vi "Machine - Config File.vi"(5 "Setting":bool, 6 "Action":enum16{"Write", "Read", "Read All", "Remove"}(ring), 7 "V1":bool, 8 "error in (no error)":errorcluster, 9 "Value":string[](array[string]), 10 "Key Name":string[](array[string]), 11 "IP/SN":string) -> (0 "error out":errorcluster, 3 "Value Out":cluster{"IP/SN":string, "Key Value":string[]}[](array[cluster]))   [LabVIEW 2019]
uses:
  <vilib>/Utility/config.llb/Write Key (String).vi
  <vilib>/Utility/config.llb/Read Key (String).vi
  <vilib>/httpClient/POSTBuffer.vi
  <vilib>/Utility/config.llb/NI_LVConfig.lvlib
  <vilib>/httpClient/LabVIEWHTTPClient.lvlib
panel:
  out "?":cluster{"IP/SN":string, "Key Value":string[]}={"IP/SN"="TP2-240203", "Key Value"=["COM6", "TEST2", "0", "N/A"]}
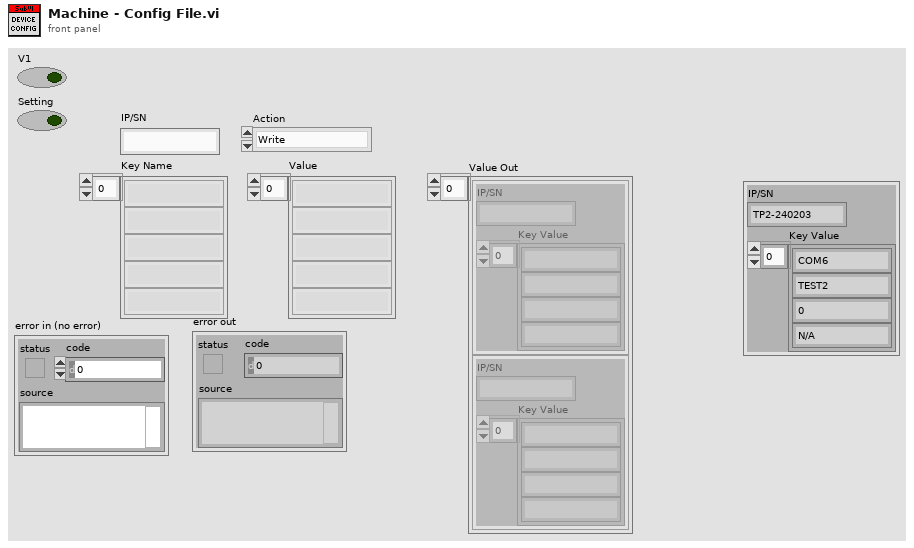
[diagram p1: front panel]
types:
  T1 = cluster{"action":string, "SNIP":string, "port":string, "devicename":string, "status":string, "type":string, "id":string}
  T2 = cluster{"IP Address":string, "Key Value":string[]}
  T3 = cluster{"status":string, "data":cluster{"SNIP":string, "port":string, "devicename":string, "status":string, "type":string, "delete":string, "id":string}[]}
  T4 = cluster{"action":string, "SNIP":string, "port":string, "devicename":string, "status":string, "type":string}
  T5 = typedef "NI_LVConfig.lvlib/Config Data RefNum.ctl" = refnum<k1>
  T6 = typedef "LabVIEWHTTPClient.lvlib/ClientHandle.ctl" = refnum<k1>
  T7 = cluster{"SNIP":string, "port":string, "devicename":string, "status":string, "type":string, "delete":string, "id":string}[]
  T8 = cluster{"SNIP":string, "port":string, "devicename":string, "status":string, "type":string, "delete":string, "id":string}
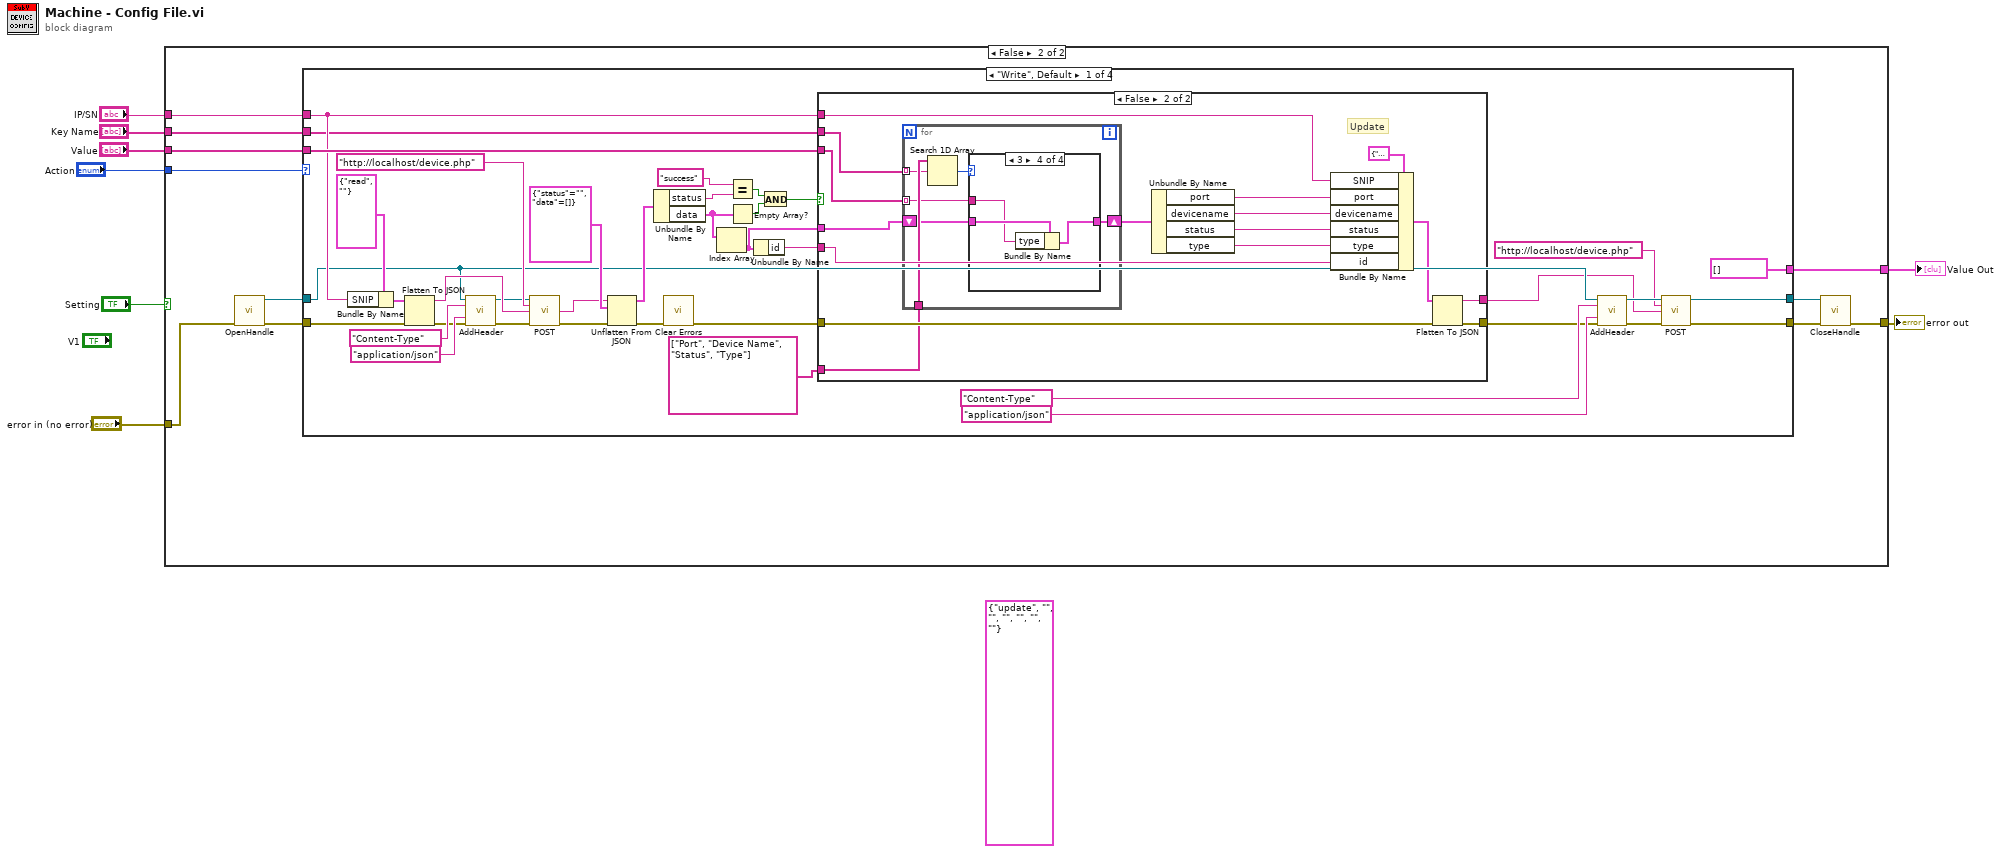
[diagram p0: block diagram]
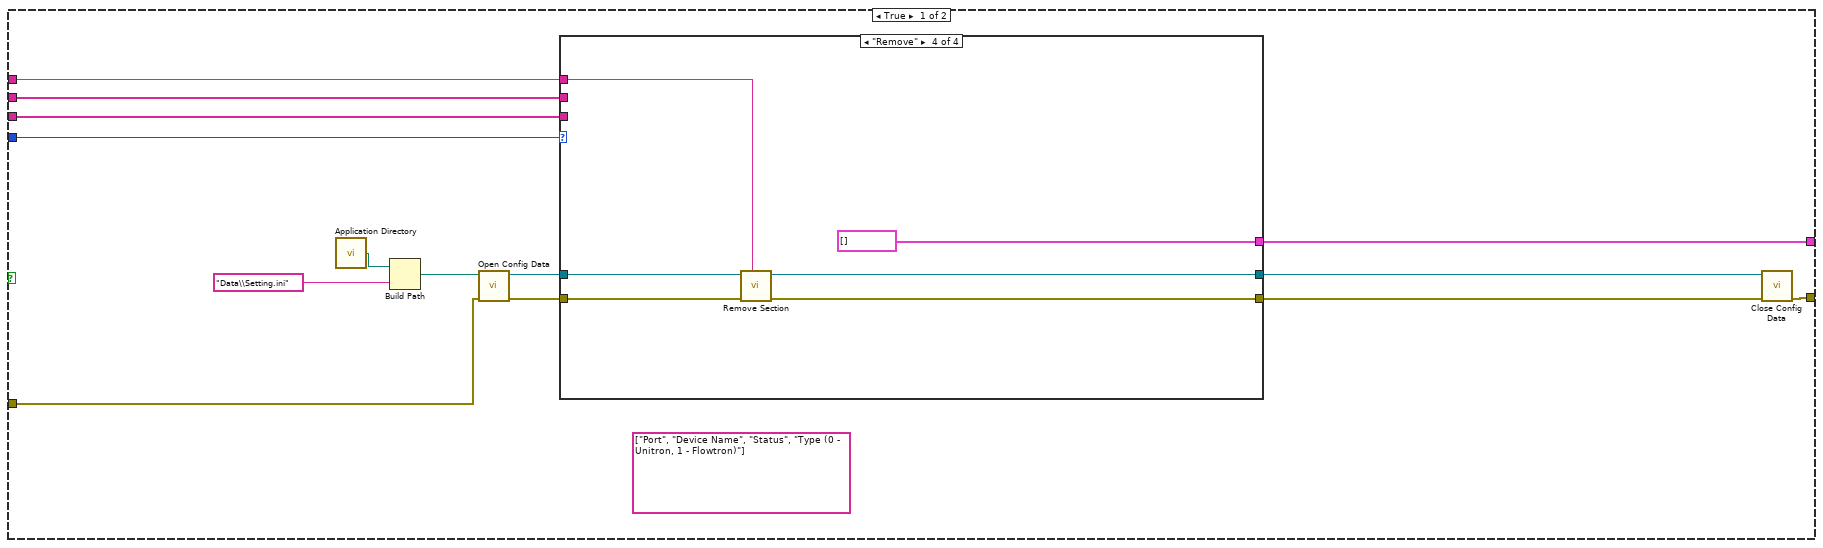
[diagram p2: hidden frame]
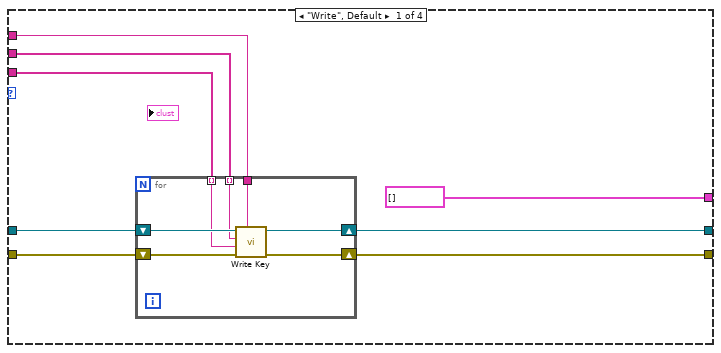
[diagram p3: hidden frame]
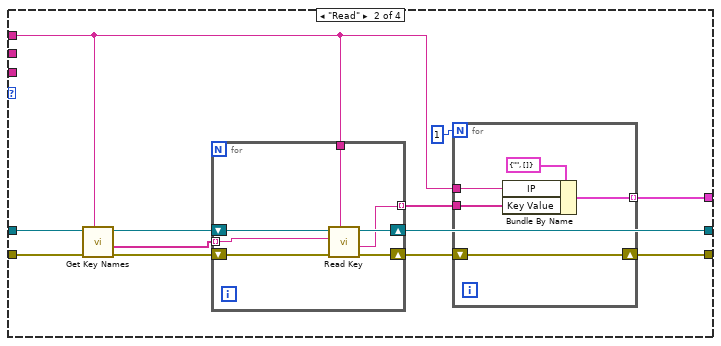
[diagram p4: hidden frame]
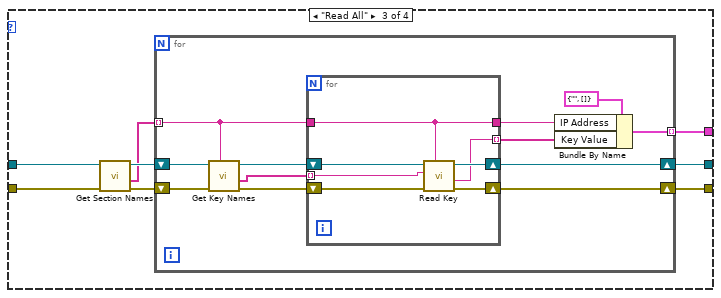
[diagram p5: hidden frame]
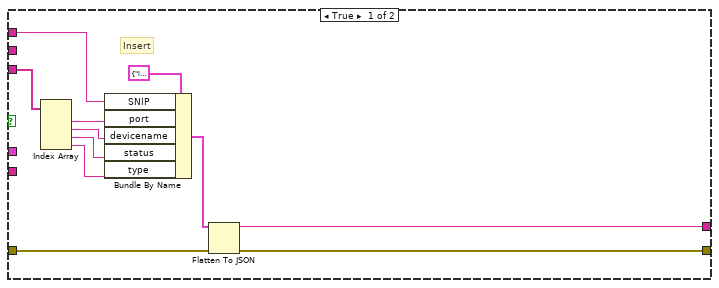
[diagram p6: hidden frame]
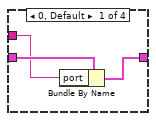
[diagram p7: hidden frame]
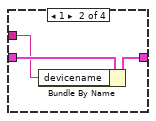
[diagram p8: hidden frame]
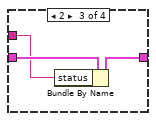
[diagram p9: hidden frame]
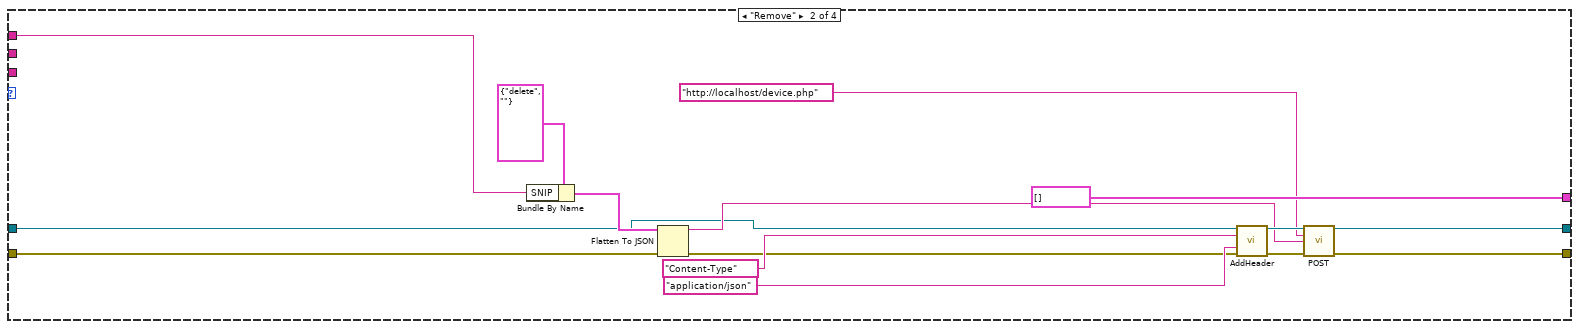
[diagram p10: hidden frame]
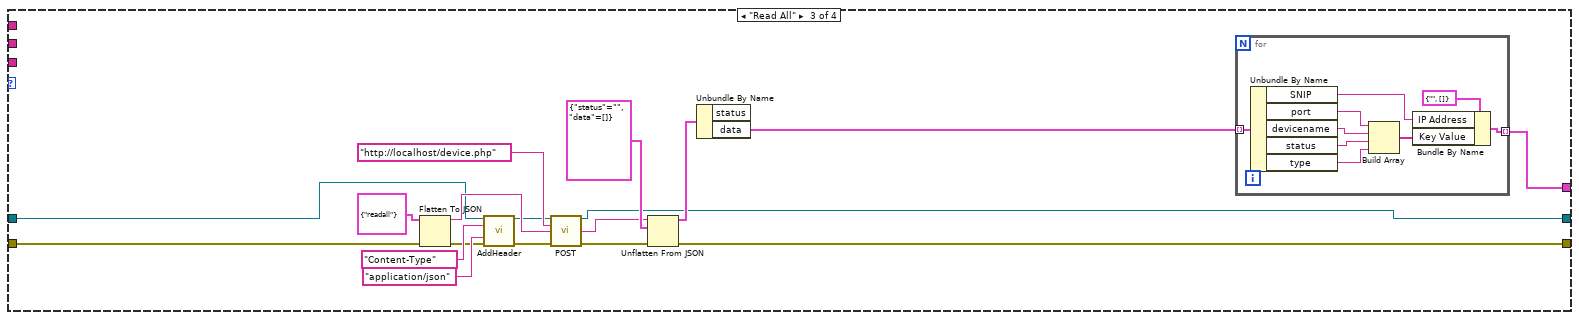
[diagram p11: hidden frame]
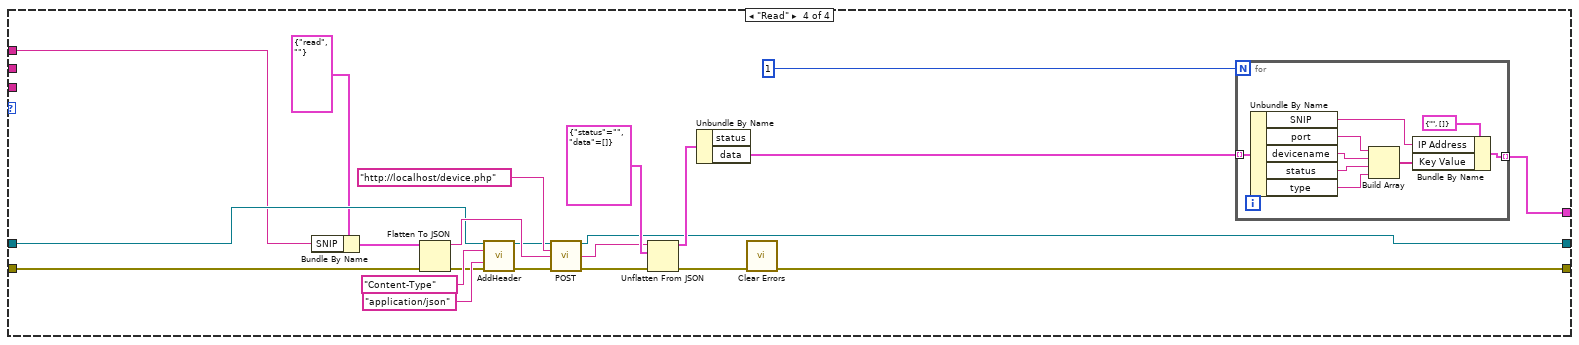
[diagram p12: hidden frame]
diagram:
  (unwired) T1 {"action"="update", "SNIP"="", "port"="", "devicename"="", "status"="", "type"="", "id"=""}
  n1 = case shown="False" "Setting" {
    tunnel: [w16 w95] -> w8
    tunnel: [w14 w105] -> w7
    tunnel: "error in (no error)" -> [w13 w98]
    tunnel: "Action" -> [w12 w104]
    tunnel: "Value" -> [w11 w103]
    tunnel: "Key Name" -> [w10 w102]
    tunnel: "IP/SN" -> [w9 w101]
    frame True {
      (unwired) string[] ["Port", "Device Name", "Status", "Type (0 - Unitron, 1 - Flowtron)"] ("Key Name")
      n2 = call <vilib>:"Application Directory.vi"() -> ("Application Directory"=w22:path)
      n3 = Build Path(base path=w22, name or relative path="Data\\Setting.ini") -> (appended path=w15:path)
      n4 = call <vilib>:"Open Config Data.vi"("error in (no error)"=w13, "configuration file path"=w15) -> ("error out"=w20:errorcluster, "refnum"=w19:T5)  [unwired: 7 in, 1 out]
      n5 = case shown="\"Remove\"" w12 {
        tunnel: w20 -> [w30 w41 w66 w92]
        tunnel: w19 -> [w29 w42 w65 w94]
        tunnel: [w28 w49 w68 w93] -> w18
        tunnel: [w27 w45 w69 w91] -> w17
        tunnel: w11 -> [w26 _ _ _]
        tunnel: w10 -> [w25 _ _ _]
        tunnel: w9 -> [w24 w39 _ w90]
        tunnel: [cluster{"Station Name":string, "Key":string[]}[] [] w47 w67 cluster{"Station Name":string, "Key":string[]}[] []] -> w14
        frame "Write", Default {
          n6 = for {
            shift-right: [w34] -> w27
            shift-left: w30 -> [w37]
            shift-right: [w35] -> w28
            shift-left: w29 -> [w36]
            tunnel: w24 -> [w33]
            tunnel: w25 -> [w32] mode=indexing
            tunnel: w26 -> [w31] mode=indexing
            n7 = call-poly <vilib>:"Write Key.vi"("section"=w33, "error in (no error)"=w37, "value"=w31, "key"=w32, "refnum"=w36) -> ("error out"=w34:errorcluster, "refnum out"=w35:T5)  [unwired: 4 in, 1 out]
          }
        }
        frame "Read" {
          n8 = call <vilib>:"Get Key Names.vi"("section"=w39, "error in (no error)"=w41, "refnum"=w42) -> ("error out"=w40:errorcluster, "key names"=w38:string[], "refnum out"=w43:T5)  [unwired: 5 in, 1 out]
          n9 = for {
            tunnel: w39 -> [w57]
            shift-right: [w58] -> w49
            shift-left: w43 -> [w61]
            shift-right: [w59] -> w44
            shift-left: w40 -> [w60]
            tunnel: [w56] -> w48 mode=indexing
            tunnel: w38 -> [w55] mode=indexing
            n10 = call-poly <vilib>:"Read Key.vi"("section"=w57, "error in (no error)"=w60, "key"=w55, "refnum"=w61) -> ("error out"=w59:errorcluster, "value"=w56:string, "refnum out"=w58:T5)  [unwired: 4 in, 1 out]
          }
          n11 = for {
            N: 1 -> [_]
            tunnel: w39 -> [w53]
            tunnel: w48 -> [w52]
            tunnel: [w51] -> w47 mode=indexing
            shift-right: [w50] -> w45
            shift-left: w44 -> [w50]
            n12 = Bundle By Name(cluster=cluster{"IP":string, "Key Value":string[]} {"IP"="", "Key Value"=[]}, "IP"=w53, "Key Value"=w52) -> (w51:cluster{"IP":string, "Key Value":string[]})
          }
        }
        frame "Read All" {
          n13 = call <vilib>:"Get Section Names.vi"("error in (no error)"=w66, "refnum"=w65) -> ("error out"=w64:errorcluster, "section names"=w62:string[], "refnum out"=w63:T5)  [unwired: 7 in]
          n14 = for {
            tunnel: [w70] -> w67 mode=indexing
            shift-right: [w81] -> w69
            shift-left: w64 -> [w79]
            shift-right: [w80] -> w68
            shift-left: w63 -> [w77]
            tunnel: w62 -> [w74] mode=indexing
            n15 = call <vilib>:"Get Key Names.vi"("section"=w74, "error in (no error)"=w79, "refnum"=w77) -> ("error out"=w78:errorcluster, "key names"=w75:string[], "refnum out"=w76:T5)  [unwired: 5 in, 1 out]
            n16 = for {
              shift-right: [w85] -> w80
              shift-left: w76 -> [w88]
              shift-right: [w86] -> w81
              shift-left: w78 -> [w87]
              tunnel: [w84] -> w71 mode=indexing
              tunnel: w75 -> [w83] mode=indexing
              tunnel: w74 -> [w82]
              tunnel: [w82] -> w72
              n17 = call-poly <vilib>:"Read Key.vi"("section"=w82, "error in (no error)"=w87, "key"=w83, "refnum"=w88) -> ("error out"=w86:errorcluster, "value"=w84:string, "refnum out"=w85:T5)  [unwired: 4 in, 1 out]
            }
            n18 = Bundle By Name(cluster=T2 {"IP Address"="", "Key Value"=[]}, "IP Address"=w72, "Key Value"=w71) -> (w70:T2)
          }
        }
        frame "Remove" {
          n19 = call <vilib>:"Remove Section.vi"("section"=w90, "error in (no error)"=w92, "refnum"=w94) -> ("error out"=w91:errorcluster, "refnum out"=w93:T5)  [unwired: 6 in, 1 out]
        }
      }
      n20 = call <vilib>:"Close Config Data.vi"("error in (no error)"=w17, "refnum"=w18) -> ("error out"=w16:errorcluster)  [unwired: 8 in, 1 out]
    }
    frame False {
      n21 = call <vilib>:"OpenHandle.vi"("error in (no error)"=w98) -> ("client handle out"=w100:T6, "error out"=w99:errorcluster)  [unwired: 13 in]
      n22 = case shown="\"Write\", Default" w104 {
        tunnel: w99 -> [w121 w195 w210 w242]
        tunnel: w103 -> [w138 _ _ _]
        tunnel: w102 -> [w108 _ _ _]
        tunnel: w101 -> [w120 w190 _ w234]
        tunnel: [cluster{"Station Name":string, "Key":string[]}[] [] cluster{"Station Name":string, "Key":string[]}[] [] w222 w253] -> w105
        tunnel: w100 -> [w119 w194 w206 w238]
        tunnel: [w137 w192 w207 w239] -> w97
        tunnel: [w136 w191 w208 w232] -> w96
        frame "Write", Default {
          n23 = Bundle By Name(cluster=cluster{"action":string, "SNIP":string} {"action"="read", "SNIP"=""}, "SNIP"=w120) -> (w122:cluster{"action":string, "SNIP":string})
          n24 = Flatten To JSON(anything=w122, error in (no error)=w121) -> (JSON string=w133:string, 11:w126:errorcluster)  [unwired: 1 in]
          n25 = call <vilib>:"AddHeader.vi"("client handle"=w119, "header"="Content-Type", "value"="application/json", "error in (no error)"=w126) -> ("client handle out"=w129:T6, "error out"=w128:errorcluster)  [unwired: 10 in]
          n26 = call-poly <vilib>:"POST.vi"("client handle"=w129, "url"="http://localhost/device.php", "buffer"=w133, "error in (no error)"=w128) -> ("body"=w127:string, "error out"=w125:errorcluster)  [unwired: 8 in, 2 out]
          n27 = Unflatten From JSON(JSON string=w127, type and defaults=T3 {"status"="", "data"=[]}, error in (no error)=w125) -> (value=w134:T3, error out=w124:errorcluster)  [unwired: 4 in]
          n28 = Unbundle By Name(w134) -> ("status"=w117:string, "data"=w118:T7)
          n29 = call <vilib>:"Clear Errors.vi"("error in (no error)"=w124) -> ("error out"=w112:errorcluster)  [unwired: 5 in, 1 out]
          n30 = Index Array(array=w118) -> (element=w106:T8)  [unwired: 1 in]
          n31 = Equal?(x="success", y=w117) -> (x = y?=w115:bool)
          n32 = Empty Array?(array=w118) -> (empty?=w114:bool)
          n33 = Unbundle By Name(w106) -> ("id"=w109:string)
          n34 = And(x=w115, y=w114) -> (x .and. y?=w113:bool)
          n35 = case shown="False" w113 {
            tunnel: w138 -> [w154 w163]
            tunnel: w120 -> [w150 w171]
            tunnel: w112 -> [w148 w170]
            tunnel: [w147 w169] -> w111
            tunnel: [w146 w168] -> w110
            tunnel: w109 -> [_ w166]
            tunnel: w108 -> [_ w165]
            tunnel: string[] ["Port", "Device Name", "Status", "Type"] ("Key Name") -> [_ w164]
            tunnel: w106 -> [_ w162]
            frame True {
              # "Insert"
              n36 = Index Array(array=w154) -> (element #1=w153:string, element #2=w145:string, element #3=w152:string, element #4=w151:string)  [unwired: 4 in]
              n37 = Bundle By Name(cluster=T4 {"action"="insert", "SNIP"="", "port"="", "devicename"="", "status"="", "type"=""}, "SNIP"=w150, "port"=w153, "devicename"=w145, "status"=w152, "type"=w151) -> (w149:T4)
              n38 = Flatten To JSON(anything=w149, error in (no error)=w148) -> (JSON string=w146:string, 11:w147:errorcluster)  [unwired: 1 in]
            }
            frame False {
              # "Update"
              n39 = for {
                tunnel: w165 -> [w176] mode=indexing
                tunnel: w164 -> [w177]
                tunnel: w163 -> [w174] mode=indexing
                shift-right: [w172] -> w160
                shift-left: w162 -> [w173]
                n40 = Search 1D Array(1D array=w177, element=w176) -> (index of element=w175:i32)  [unwired: 1 in]
                n41 = case shown="3" w175 {
                  tunnel: w174 -> [w179 w182 w185 w188]
                  tunnel: w173 -> [w180 w183 w186 w189]
                  tunnel: [w178 w181 w184 w187] -> w172
                  frame 0, Default {
                    n42 = Bundle By Name(cluster=w180, "port"=w179) -> (w178:T8)
                  }
                  frame 1 {
                    n43 = Bundle By Name(cluster=w183, "devicename"=w182) -> (w181:T8)
                  }
                  frame 2 {
                    n44 = Bundle By Name(cluster=w186, "status"=w185) -> (w184:T8)
                  }
                  frame 3 {
                    n45 = Bundle By Name(cluster=w189, "type"=w188) -> (w187:T8)
                  }
                }
              }
              n46 = Unbundle By Name(w160) -> ("port"=w159:string, "devicename"=w158:string, "status"=w157:string, "type"=w156:string)
              n47 = Bundle By Name(cluster=T1 {"action"="update", "SNIP"="", "port"="", "devicename"="", "status"="", "type"="", "id"=""}, "SNIP"=w171, "port"=w159, "devicename"=w158, "status"=w157, "type"=w156, "id"=w166) -> (w167:T1)
              n48 = Flatten To JSON(anything=w167, error in (no error)=w170) -> (JSON string=w168:string, 11:w169:errorcluster)  [unwired: 1 in]
            }
          }
          n49 = call <vilib>:"AddHeader.vi"("client handle"=w119, "header"="Content-Type", "value"="application/json", "error in (no error)"=w111) -> ("client handle out"=w142:T6, "error out"=w143:errorcluster)  [unwired: 10 in]
          n50 = call-poly <vilib>:"POST.vi"("client handle"=w142, "url"="http://localhost/device.php", "buffer"=w110, "error in (no error)"=w143) -> ("client handle out"=w137:T6, "error out"=w136:errorcluster)  [unwired: 8 in, 2 out]
        }
        frame "Remove" {
          n51 = Bundle By Name(cluster=cluster{"action":string, "SNIP":string} {"action"="delete", "SNIP"=""}, "SNIP"=w190) -> (w198:cluster{"action":string, "SNIP":string})
          n52 = Flatten To JSON(anything=w198, error in (no error)=w195) -> (JSON string=w196:string, 11:w193:errorcluster)  [unwired: 1 in]
          n53 = call <vilib>:"AddHeader.vi"("client handle"=w194, "header"="Content-Type", "value"="application/json", "error in (no error)"=w193) -> ("client handle out"=w202:T6, "error out"=w203:errorcluster)  [unwired: 10 in]
          n54 = call-poly <vilib>:"POST.vi"("client handle"=w202, "url"="http://localhost/device.php", "buffer"=w196, "error in (no error)"=w203) -> ("client handle out"=w192:T6, "error out"=w191:errorcluster)  [unwired: 8 in, 2 out]
        }
        frame "Read All" {
          n55 = Flatten To JSON(anything=cluster{"action":string} {"action"="readall"}, error in (no error)=w210) -> (JSON string=w219:string, 11:w211:errorcluster)  [unwired: 1 in]
          n56 = call <vilib>:"AddHeader.vi"("client handle"=w206, "header"="Content-Type", "value"="application/json", "error in (no error)"=w211) -> ("client handle out"=w215:T6, "error out"=w214:errorcluster)  [unwired: 10 in]
          n57 = call-poly <vilib>:"POST.vi"("client handle"=w215, "url"="http://localhost/device.php", "buffer"=w219, "error in (no error)"=w214) -> ("client handle out"=w207:T6, "body"=w213:string, "error out"=w209:errorcluster)  [unwired: 8 in, 1 out]
          n58 = Unflatten From JSON(JSON string=w213, type and defaults=T3 {"status"="", "data"=[]}, error in (no error)=w209) -> (value=w220:T3, error out=w208:errorcluster)  [unwired: 4 in]
          n59 = Unbundle By Name(w220) -> ("data"=w205:T7)  [unwired: 1 out]
          n60 = for {
            tunnel: [w230] -> w222 mode=indexing
            tunnel: w205 -> [w229] mode=indexing
            n61 = Unbundle By Name(w229) -> ("SNIP"=w228:string, "port"=w227:string, "devicename"=w226:string, "status"=w223:string, "type"=w225:string)
            n62 = Build Array(w227, w226, w223, w225) -> (w224:string[])
            n63 = Bundle By Name(cluster=T2 {"IP Address"="", "Key Value"=[]}, "IP Address"=w228, "Key Value"=w224) -> (w230:T2)
          }
        }
        frame "Read" {
          n64 = Bundle By Name(cluster=cluster{"action":string, "SNIP":string} {"action"="read", "SNIP"=""}, "SNIP"=w234) -> (w235:cluster{"action":string, "SNIP":string})
          n65 = Flatten To JSON(anything=w235, error in (no error)=w242) -> (JSON string=w250:string, 11:w243:errorcluster)  [unwired: 1 in]
          n66 = call <vilib>:"AddHeader.vi"("client handle"=w238, "header"="Content-Type", "value"="application/json", "error in (no error)"=w243) -> ("client handle out"=w246:T6, "error out"=w245:errorcluster)  [unwired: 10 in]
          n67 = call-poly <vilib>:"POST.vi"("client handle"=w246, "url"="http://localhost/device.php", "buffer"=w250, "error in (no error)"=w245) -> ("client handle out"=w239:T6, "body"=w244:string, "error out"=w241:errorcluster)  [unwired: 8 in, 1 out]
          n68 = Unflatten From JSON(JSON string=w244, type and defaults=T3 {"status"="", "data"=[]}, error in (no error)=w241) -> (value=w251:T3, error out=w240:errorcluster)  [unwired: 4 in]
          n69 = Unbundle By Name(w251) -> ("data"=w237:T7)  [unwired: 1 out]
          n70 = call <vilib>:"Clear Errors.vi"("error in (no error)"=w240) -> ("error out"=w232:errorcluster)  [unwired: 5 in, 1 out]
          n71 = for {
            N: 1 -> [_]
            tunnel: [w261] -> w253 mode=indexing
            tunnel: w237 -> [w260] mode=indexing
            n72 = Unbundle By Name(w260) -> ("SNIP"=w259:string, "port"=w258:string, "devicename"=w257:string, "status"=w254:string, "type"=w256:string)
            n73 = Build Array(w258, w257, w254, w256) -> (w255:string[])
            n74 = Bundle By Name(cluster=T2 {"IP Address"="", "Key Value"=[]}, "IP Address"=w259, "Key Value"=w255) -> (w261:T2)
          }
        }
      }
      n75 = call <vilib>:"CloseHandle.vi"("client handle"=w97, "error in (no error)"=w96) -> ("error out"=w95:errorcluster)  [unwired: 13 in]
    }
  }
  "error out" <- w8
  "Value Out" <- w7
